vi "Main.vi"   [LabVIEW 2016]
uses:
  Simulation Interface/Simulation Interface.lvclass
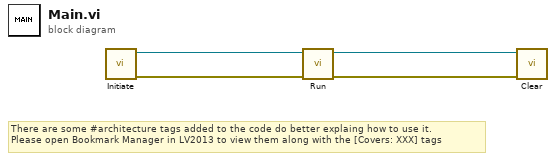
[diagram p0: block diagram]
diagram:
  # "There are some #architecture tags added to the code do better explaing how to use it.\nPlease open Bookmark Manager in LV2013 to view them along with the [Covers: XXX] tags"
  n1 = call "Initiate.vi"() -> ("error out"=w3:errorcluster, "Simulation Interface out"=w4:refnum<class "Simulation Interface.lvclass">)  [unwired: 10 in]
  n2 = call "Run.vi"("error in (no error)"=w3, "Simulation Interface in"=w4) -> ("error out"=w1:errorcluster, "Simulation Interface out"=w2:refnum<class "Simulation Interface.lvclass">)  [unwired: 8 in]
  n3 = call "Clear.vi"("error in (no error)"=w1, "Simulation Interface in"=w2) -> ()  [unwired: 9 in, 1 out]
